vi "Get Environment Variable Value.vi"(0 "Environment Variable":string) -> (1 "Value":string, 2 "error out":errorcluster)   [LabVIEW 2016]
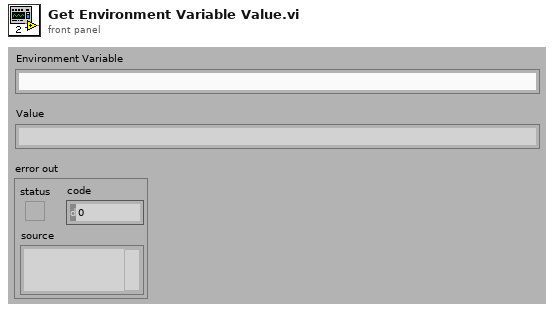
[diagram p1: front panel]
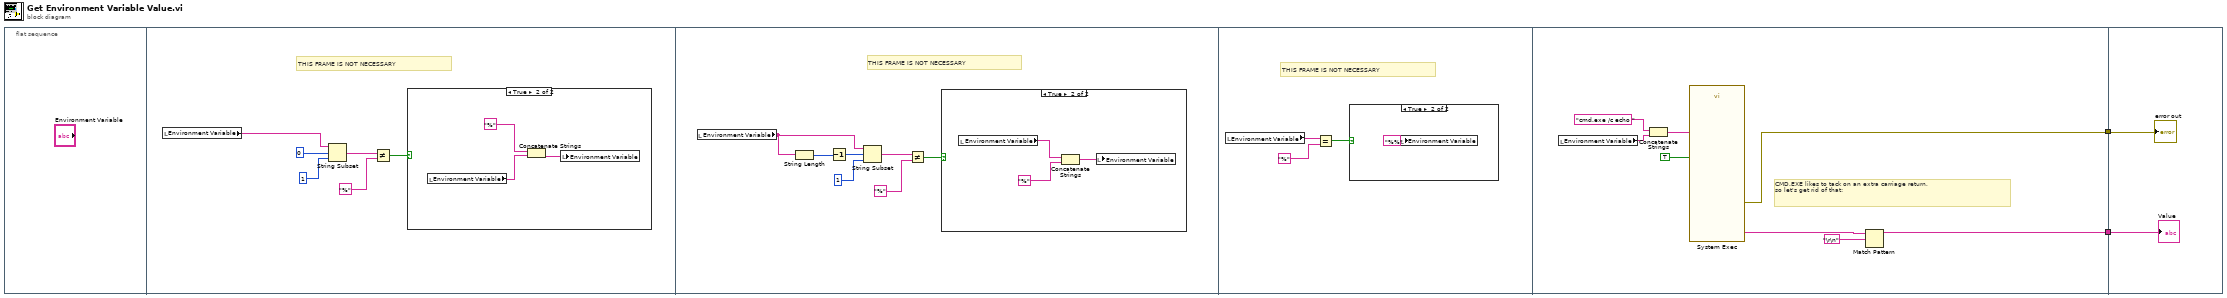
[diagram p0: block diagram]
diagram:
  n1 = flat-sequence {
    tunnel: [w27] -> w2
    tunnel: [w26] -> w1
    tunnel: w2 -> [w35]
    tunnel: w1 -> [w34]
    frame #0 {
    }
    frame #1 {
      # "THIS FRAME IS NOT NECESSARY"
      n2 = local read "Environment Variable"() -> (w7:string)
      n3 = String Subset(string=w7, offset (0)=0, length (rest)=1 ("length (rest)")) -> (substring=w6:string)
      n4 = Not Equal?(x=w6, y="%") -> (x != y?=w4:bool)
      n5 = case shown="True" w4 {
        frame False {
        }
        frame True {
          n6 = local read "Environment Variable"() -> (w11:string)
          n7 = Concatenate Strings("%" ("string"), w11) -> (w10:string)
          n8 = local write "Environment Variable"(w10) -> ()
        }
      }
    }
    frame #2 {
      # "THIS FRAME IS NOT NECESSARY"
      n9 = local read "Environment Variable"() -> (w15:string)
      n10 = String Length(string=w15) -> (length=w12:i32)
      n11 = Decrement(x=w12) -> (x-1=w13:i32)
      n12 = String Subset(string=w15, offset (0)=w13, length (rest)=1 ("length (rest)")) -> (substring=w16:string)
      n13 = Not Equal?(x=w16, y="%") -> (x != y?=w18:bool)
      n14 = case shown="True" w18 {
        frame False {
        }
        frame True {
          n15 = local read "Environment Variable"() -> (w21:string)
          n16 = Concatenate Strings(w21, "%" ("string")) -> (w19:string)
          n17 = local write "Environment Variable"(w19) -> ()
        }
      }
    }
    frame #3 {
      # "THIS FRAME IS NOT NECESSARY"
      n18 = local read "Environment Variable"() -> (w24:string)
      n19 = Equal?(x=w24, y="%") -> (x = y?=w23:bool)
      n20 = case shown="True" w23 {
        frame False {
        }
        frame True {
          n21 = local write "Environment Variable"("%%" ("Environment Variable")) -> ()
        }
      }
    }
    frame #4 {
      # "CMD.EXE likes to tack on an extra carriage return,\nso let's get rid of that:"
      n22 = local read "Environment Variable"() -> (w31:string)
      n23 = Concatenate Strings("cmd.exe /c echo " ("command line"), w31) -> (w30:string)
      n24 = call <vilib>:"System Exec.vi"("run minimized? (F)"=TRUE, "command line"=w30) -> ("error out"=w26:errorcluster, "standard output"=w28:string)  [unwired: 6 in, 2 out]
      n25 = Match Pattern(string=w28, regular expression="\r\n") -> (before substring=w27:string)  [unwired: 1 in, 3 out]
    }
    frame #5 {
      "Value" <- w35
      "error out" <- w34
    }
  }
